vi "Set Window Position.vi"(8 "error in (no error)":errorcluster, 10 "Mouse Coordinates":T1, 11 "VI in":refnum<vi>) -> (0 "error out":errorcluster)   [LabVIEW 2019]
uses:
  <vilib>/Utility/miscctls.llb/LVPoint32TypeDef.ctl
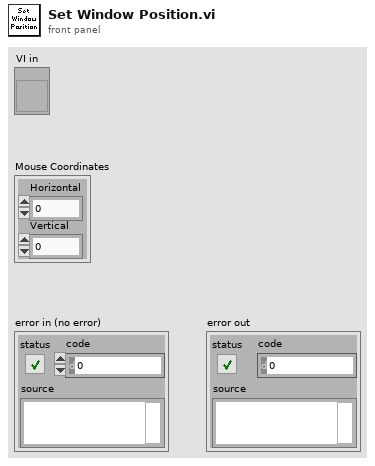
[diagram p1: front panel]
types:
  T1 = typedef "LVPoint32TypeDef.ctl" = cluster{"Horizontal":i32, "Vertical":i32}
  T2 = enum32{"Invalid", "Standard", "Closed", "Hidden", "Minimized", "Maximized"}
  T3 = typedef "LVRectTypeDef.ctl" = cluster{"Left":i16, "Top":i16, "Right":i16, "Bottom":i16}
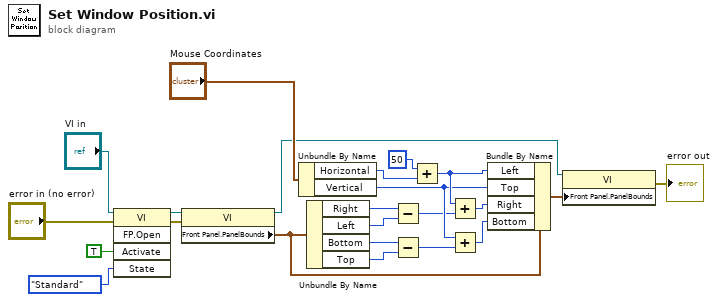
[diagram p0: block diagram]
diagram:
  n1 = invoke class="VI" method="FP.Open"(reference="VI in", error in="error in (no error)", "Activate"=TRUE ("Activate?"), "State"=T2."Standard") -> (reference out=w3:refnum<vi>, error out=w4:errorcluster)  [unwired: 1 in, 3 out]
  n2 = property class="VI"(reference=w3, error in=w4) -> (reference out=w8:refnum<vi>, "Front Panel.PanelBounds"=w11:T3)  [unwired: 1 out]
  n3 = Unbundle By Name("Mouse Coordinates") -> ("Horizontal"=w17:i32, "Vertical"=w20:i32)
  n4 = Unbundle By Name(w11) -> ("Right"=w12:i16, "Left"=w13:i16, "Bottom"=w14:i16, "Top"=w15:i16)
  n5 = Subtract(x=w12, y=w13) -> (x-y=w16:i16)
  n6 = Subtract(x=w14, y=w15) -> (x-y=w19:i16)
  n7 = Add(x=50, y=w17) -> (x+y=w22:i32)
  n8 = Add(x=w22, y=w16) -> (x+y=w18:i32)
  n9 = Add(x=w20, y=w19) -> (x+y=w21:i32)
  n10 = Bundle By Name(cluster=w11, "Left"=w22, "Top"=w20, "Right"=w18, "Bottom"=w21) -> (w9:T3)
  n11 = property class="VI"(reference=w8, "Front Panel.PanelBounds"=w9) -> (error out=→"error out":errorcluster)  [unwired: 1 in, 1 out]
